vi "readLogForceActuatorSafetyChecks.vi"(8 "error in (no error)":errorcluster, 10 "Parser":refnum<class "U8ArrayParserAutoIndexing.lvclass">, 11 "M1M3SAL in":refnum<class "M1M3SAL.lvclass">) -> (0 "error out":errorcluster, 2 "EventForceActuatorSafetyChecks":variant, 3 "M1M3SAL out":refnum<class "M1M3SAL.lvclass">)   [LabVIEW 2016, in "M1M3SupportCommunicator.lvlib" / "M1M3SAL.lvclass"]
uses:
  M1M3SAL.lvclass
  Common_RT_Utilities/U8ArrayParserAutoIndexing/U8ArrayParserAutoIndexing.lvclass
  DataTypes/Topics/EventForceActuatorSafetyChecks.ctl
  DataTypes/Topics/Parts/Timestamp.ctl
  DataTypes/Topics/M1M3SupportTopics.lvlib
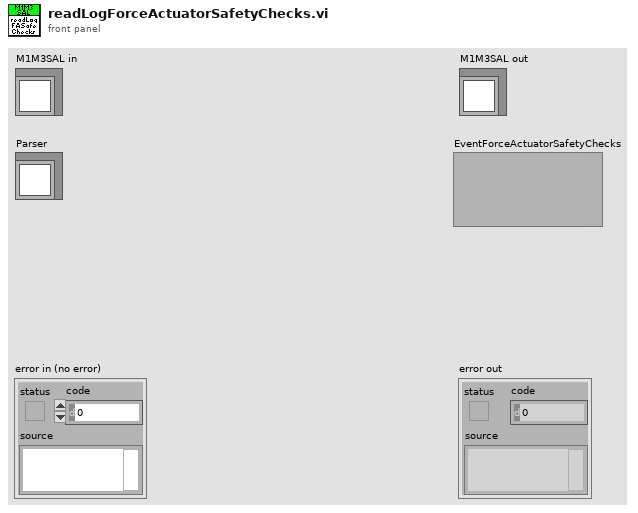
[diagram p1: front panel]
types:
  T1 = typedef "M1M3SupportTopics.lvlib/EventForceActuatorSafetyChecks.ctl" = cluster{"Timestamp":T2, "AllInSafetyLimit":bool, "SafetyLimitOk":bool[], "MirrorWeightOk":bool, "XMomentOk":bool, "YMomentOk":bool, "AllNeighborsOk":bool, "NeighborsOk":bool[], "MagnitudeOk":bool, "AllGlobalBendingOk":bool, "GlobalBendingOk":bool[], "FollowingErrorOk":bool, "AxialFollowingErrorOk":bool[], "LateralFollowingErrorOk":bool[], "AOSNetForceOk":bool, "AllElevationForcesOk":bool, "ElevationForcesOk":bool[], "AllAzimuthForcesOk":bool, "AzimuthForcesOk":bool[], "AllThermalForcesOk":bool, "ThermalForcesOk":bool[], "AllAOSForcesOk":bool, "AOSForcesOk":bool[]}
  T2 = typedef "M1M3SupportTopics.lvlib/Timestamp.ctl" = dbl
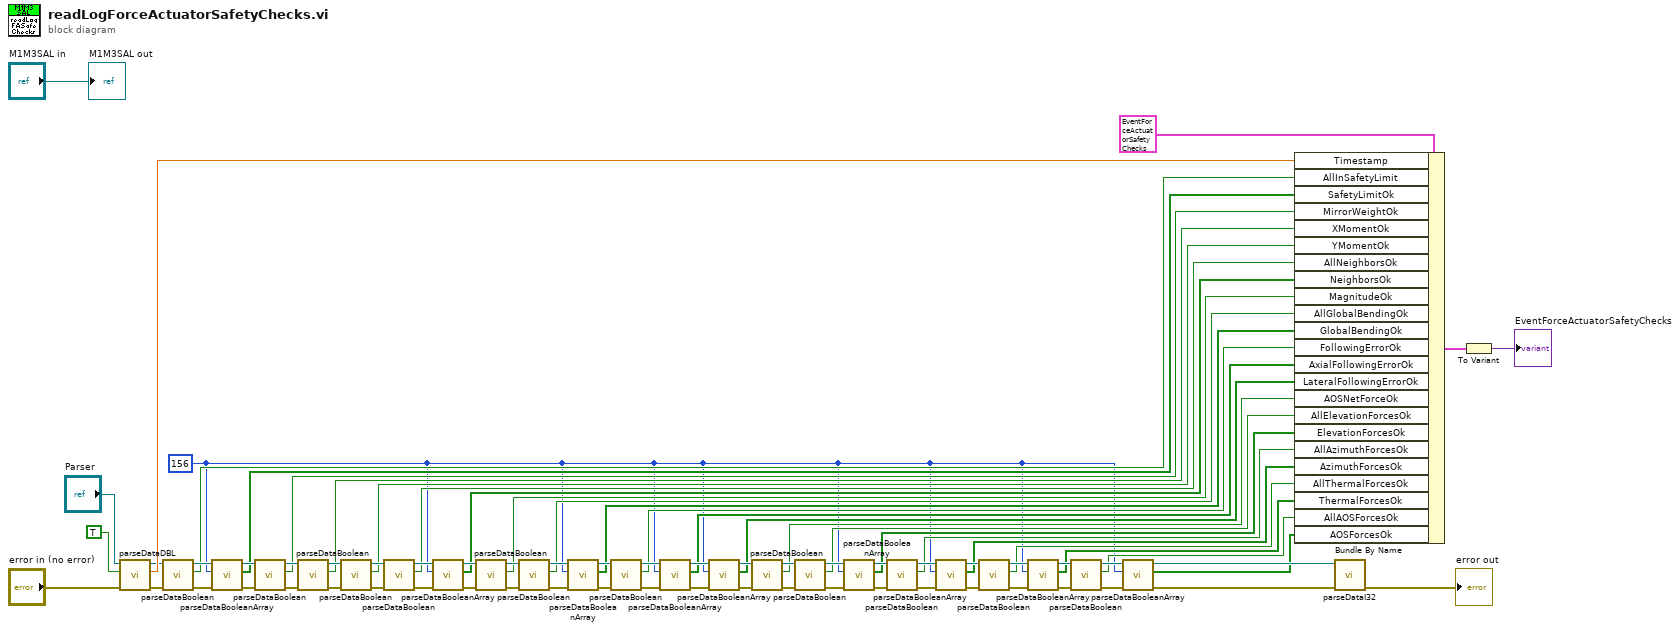
[diagram p0: block diagram]
diagram:
  w1 = 156 ("Length")
  n1 = call "parseDataDBL.vi"("error in (no error)"="error in (no error)", "OverrideSwapBytes"=TRUE, "U8ArrayParserAutoIndexing in"="Parser") -> ("error out"=w69:errorcluster, "Data"=w71:dbl, "U8ArrayParserAutoIndexing out"=w68:refnum<class "U8ArrayParserAutoIndexing.lvclass">)  [unwired: 6 in]
  n2 = call "parseDataBoolean.vi"("error in (no error)"=w69, "U8ArrayParserAutoIndexing in"=w68) -> ("error out"=w67:errorcluster, "Data"=w37:bool, "U8ArrayParserAutoIndexing out"=w66:refnum<class "U8ArrayParserAutoIndexing.lvclass">)  [unwired: 7 in]
  n3 = call "parseDataBooleanArray.vi"("error in (no error)"=w67, "Length"=w1, "U8ArrayParserAutoIndexing in"=w66) -> ("error out"=w65:errorcluster, "Data"=w36:bool[], "U8ArrayParserAutoIndexing out"=w64:refnum<class "U8ArrayParserAutoIndexing.lvclass">)  [unwired: 6 in]
  n4 = call "parseDataBoolean.vi"("error in (no error)"=w65, "U8ArrayParserAutoIndexing in"=w64) -> ("error out"=w63:errorcluster, "Data"=w35:bool, "U8ArrayParserAutoIndexing out"=w62:refnum<class "U8ArrayParserAutoIndexing.lvclass">)  [unwired: 7 in]
  n5 = call "parseDataBoolean.vi"("error in (no error)"=w63, "U8ArrayParserAutoIndexing in"=w62) -> ("error out"=w61:errorcluster, "Data"=w34:bool, "U8ArrayParserAutoIndexing out"=w60:refnum<class "U8ArrayParserAutoIndexing.lvclass">)  [unwired: 7 in]
  n6 = call "parseDataBoolean.vi"("error in (no error)"=w61, "U8ArrayParserAutoIndexing in"=w60) -> ("error out"=w59:errorcluster, "Data"=w33:bool, "U8ArrayParserAutoIndexing out"=w58:refnum<class "U8ArrayParserAutoIndexing.lvclass">)  [unwired: 7 in]
  n7 = call "parseDataBoolean.vi"("error in (no error)"=w59, "U8ArrayParserAutoIndexing in"=w58) -> ("error out"=w57:errorcluster, "Data"=w32:bool, "U8ArrayParserAutoIndexing out"=w56:refnum<class "U8ArrayParserAutoIndexing.lvclass">)  [unwired: 7 in]
  n8 = call "parseDataBooleanArray.vi"("error in (no error)"=w57, "Length"=w1, "U8ArrayParserAutoIndexing in"=w56) -> ("error out"=w55:errorcluster, "Data"=w31:bool[], "U8ArrayParserAutoIndexing out"=w54:refnum<class "U8ArrayParserAutoIndexing.lvclass">)  [unwired: 6 in]
  n9 = call "parseDataBoolean.vi"("error in (no error)"=w55, "U8ArrayParserAutoIndexing in"=w54) -> ("error out"=w53:errorcluster, "Data"=w30:bool, "U8ArrayParserAutoIndexing out"=w52:refnum<class "U8ArrayParserAutoIndexing.lvclass">)  [unwired: 7 in]
  n10 = call "parseDataBoolean.vi"("error in (no error)"=w53, "U8ArrayParserAutoIndexing in"=w52) -> ("error out"=w51:errorcluster, "Data"=w29:bool, "U8ArrayParserAutoIndexing out"=w50:refnum<class "U8ArrayParserAutoIndexing.lvclass">)  [unwired: 7 in]
  n11 = call "parseDataBooleanArray.vi"("error in (no error)"=w51, "Length"=w1, "U8ArrayParserAutoIndexing in"=w50) -> ("error out"=w49:errorcluster, "Data"=w28:bool[], "U8ArrayParserAutoIndexing out"=w48:refnum<class "U8ArrayParserAutoIndexing.lvclass">)  [unwired: 6 in]
  n12 = call "parseDataBoolean.vi"("error in (no error)"=w49, "U8ArrayParserAutoIndexing in"=w48) -> ("error out"=w47:errorcluster, "Data"=w27:bool, "U8ArrayParserAutoIndexing out"=w46:refnum<class "U8ArrayParserAutoIndexing.lvclass">)  [unwired: 7 in]
  n13 = call "parseDataBooleanArray.vi"("error in (no error)"=w47, "Length"=w1, "U8ArrayParserAutoIndexing in"=w46) -> ("error out"=w45:errorcluster, "Data"=w26:bool[], "U8ArrayParserAutoIndexing out"=w44:refnum<class "U8ArrayParserAutoIndexing.lvclass">)  [unwired: 6 in]
  n14 = call "parseDataBooleanArray.vi"("error in (no error)"=w45, "Length"=w1, "U8ArrayParserAutoIndexing in"=w44) -> ("error out"=w43:errorcluster, "Data"=w25:bool[], "U8ArrayParserAutoIndexing out"=w42:refnum<class "U8ArrayParserAutoIndexing.lvclass">)  [unwired: 6 in]
  n15 = call "parseDataBoolean.vi"("error in (no error)"=w43, "U8ArrayParserAutoIndexing in"=w42) -> ("error out"=w41:errorcluster, "Data"=w24:bool, "U8ArrayParserAutoIndexing out"=w40:refnum<class "U8ArrayParserAutoIndexing.lvclass">)  [unwired: 7 in]
  n16 = call "parseDataBoolean.vi"("error in (no error)"=w41, "U8ArrayParserAutoIndexing in"=w40) -> ("error out"=w39:errorcluster, "Data"=w23:bool, "U8ArrayParserAutoIndexing out"=w38:refnum<class "U8ArrayParserAutoIndexing.lvclass">)  [unwired: 7 in]
  n17 = call "parseDataBooleanArray.vi"("error in (no error)"=w39, "Length"=w1, "U8ArrayParserAutoIndexing in"=w38) -> ("error out"=w22:errorcluster, "Data"=w8:bool[], "U8ArrayParserAutoIndexing out"=w21:refnum<class "U8ArrayParserAutoIndexing.lvclass">)  [unwired: 6 in]
  n18 = call "parseDataBoolean.vi"("error in (no error)"=w22, "U8ArrayParserAutoIndexing in"=w21) -> ("error out"=w20:errorcluster, "Data"=w7:bool, "U8ArrayParserAutoIndexing out"=w19:refnum<class "U8ArrayParserAutoIndexing.lvclass">)  [unwired: 7 in]
  n19 = call "parseDataBooleanArray.vi"("error in (no error)"=w20, "Length"=w1, "U8ArrayParserAutoIndexing in"=w19) -> ("error out"=w18:errorcluster, "Data"=w6:bool[], "U8ArrayParserAutoIndexing out"=w17:refnum<class "U8ArrayParserAutoIndexing.lvclass">)  [unwired: 6 in]
  n20 = call "parseDataBoolean.vi"("error in (no error)"=w18, "U8ArrayParserAutoIndexing in"=w17) -> ("error out"=w16:errorcluster, "Data"=w5:bool, "U8ArrayParserAutoIndexing out"=w15:refnum<class "U8ArrayParserAutoIndexing.lvclass">)  [unwired: 7 in]
  n21 = call "parseDataBooleanArray.vi"("error in (no error)"=w16, "Length"=w1, "U8ArrayParserAutoIndexing in"=w15) -> ("error out"=w11:errorcluster, "Data"=w4:bool[], "U8ArrayParserAutoIndexing out"=w12:refnum<class "U8ArrayParserAutoIndexing.lvclass">)  [unwired: 6 in]
  n22 = call "parseDataBoolean.vi"("error in (no error)"=w11, "U8ArrayParserAutoIndexing in"=w12) -> ("error out"=w14:errorcluster, "Data"=w3:bool, "U8ArrayParserAutoIndexing out"=w13:refnum<class "U8ArrayParserAutoIndexing.lvclass">)  [unwired: 7 in]
  n23 = call "parseDataBooleanArray.vi"("error in (no error)"=w14, "Length"=w1, "U8ArrayParserAutoIndexing in"=w13) -> ("error out"=w9:errorcluster, "Data"=w2:bool[], "U8ArrayParserAutoIndexing out"=w10:refnum<class "U8ArrayParserAutoIndexing.lvclass">)  [unwired: 6 in]
  n24 = Bundle By Name(cluster=T1 {"Timestamp"=0.0, "AllInSafetyLimit"=FALSE, "SafetyLimitOk"=[], "MirrorWeightOk"=FALSE, "XMomentOk"=FALSE, "YMomentOk"=FALSE, "AllNeighborsOk"=FALSE, "NeighborsOk"=[], "MagnitudeOk"=FALSE, "AllGlobalBendingOk"=FALSE, "GlobalBendingOk"=[], "FollowingErrorOk"=FALSE, "AxialFollowingErrorOk"=[], "LateralFollowingErrorOk"=[], "AOSNetForceOk"=FALSE, "AllElevationForcesOk"=FALSE, "ElevationForcesOk"=[], "AllAzimuthForcesOk"=FALSE, "AzimuthForcesOk"=[], "AllThermalForcesOk"=FALSE, "ThermalForcesOk"=[], "AllAOSForcesOk"=FALSE, "AOSForcesOk"=[]} ("EventForceActuatorSafetyChecks"), "Timestamp"=w71, "AllInSafetyLimit"=w37, "SafetyLimitOk"=w36, "MirrorWeightOk"=w35, "XMomentOk"=w34, "YMomentOk"=w33, "AllNeighborsOk"=w32, "NeighborsOk"=w31, "MagnitudeOk"=w30, "AllGlobalBendingOk"=w29, "GlobalBendingOk"=w28, "FollowingErrorOk"=w27, "AxialFollowingErrorOk"=w26, "LateralFollowingErrorOk"=w25, "AOSNetForceOk"=w24, "AllElevationForcesOk"=w23, "ElevationForcesOk"=w8, "AllAzimuthForcesOk"=w7, "AzimuthForcesOk"=w6, "AllThermalForcesOk"=w5, "ThermalForcesOk"=w4, "AllAOSForcesOk"=w3, "AOSForcesOk"=w2) -> (w77:T1)
  n25 = call "parseDataI32.vi"("error in (no error)"=w9, "U8ArrayParserAutoIndexing in"=w10) -> ("error out"=→"error out":errorcluster)  [unwired: 7 in, 2 out]
  n26 = To Variant(anything=w77) -> (Variant=→"EventForceActuatorSafetyChecks":variant)
  "M1M3SAL out" <- "M1M3SAL in"
